vi "Size2003.vi"   [LabVIEW 2013]
uses:
  <vilib>/Heliosphere Research LLC/Advanced Plotting Toolkit/Advanced Plotting Toolkit.lvlib
types:
  T1 = typedef "Advanced Plotting Toolkit.lvlib/PlotID.ctl" = i32
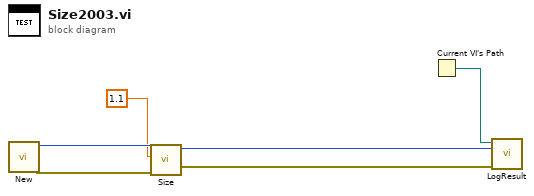
[diagram p0: block diagram]
diagram:
  n1 = call <vilib>:"New.vi"() -> ("error out"=w2:errorcluster, "Plot ID"=w5:T1)  [unwired: 10 in]
  n2 = call <vilib>:"Size.vi"("error in (no error)"=w2, "Width (pixels)"=1.1, "Plot ID"=w5) -> ("error out"=w3:errorcluster, "Plot ID Out"=w4:T1)  [unwired: 7 in]
  n3 = Current VI's Path() -> (path=w6:path)
  n4 = call "LogResult.vi"("Test Result"=w3, "Test Artifact"=w4, "VI Path"=w6) -> ()  [unwired: 9 in]
